vi "SLL DE AO LV2 Global.vi"(6 "AO value Array":dbl[](array[numeric]), 7 "AO Option":T2, 8 "error in (no error)":errorcluster, 9 "AO value":dbl, 10 "AO Channel Name Array":T1[](array[typedef]), 11 "AO Channel Name":T1) -> (0 "error out":errorcluster, 2 "Analog Output Array Value":dbl[](array[numeric]), 3 "Analog Output Line Value":dbl, 4 "Element Wrote":string)   [LabVIEW 2013]
uses:
  Controls/SLL DE AO Global Options.ctl
  Controls/SLL DE List of Analog Outputs.ctl
  Controls/SLL DE AO Command LV2Global Options.ctl
  Controls/SLL DE AO Min Max Range Checking Options.ctl
panel:
  out "Data Changed?":bool
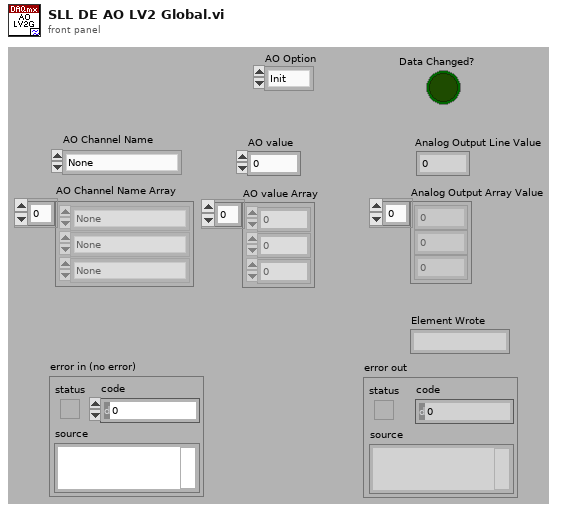
[diagram p1: front panel]
types:
  T1 = typedef "SLL DE List of Analog Outputs.ctl" = enum16{"None"}
  T2 = typedef "SLL DE AO Global Options.ctl" = enum16{"Init", "Write Line", "Write Array", "Read Line", "Read Array", "Read Full Status", "Restart AO", "Send to Safe Mode", "Stop AO"}
  T3 = typedef "SLL DE AO Command LV2Global Options.ctl" = enum16{"Init/Register Events", "Get Event Refnum", "Fire Event", "Distroy Event"}
  T4 = typedef "SLL DE AO Min Max Range Checking Options.ctl" = enum16{"Initalize Channel Range", "Check Single AO Channel", "Check Multiple AO Channels"}
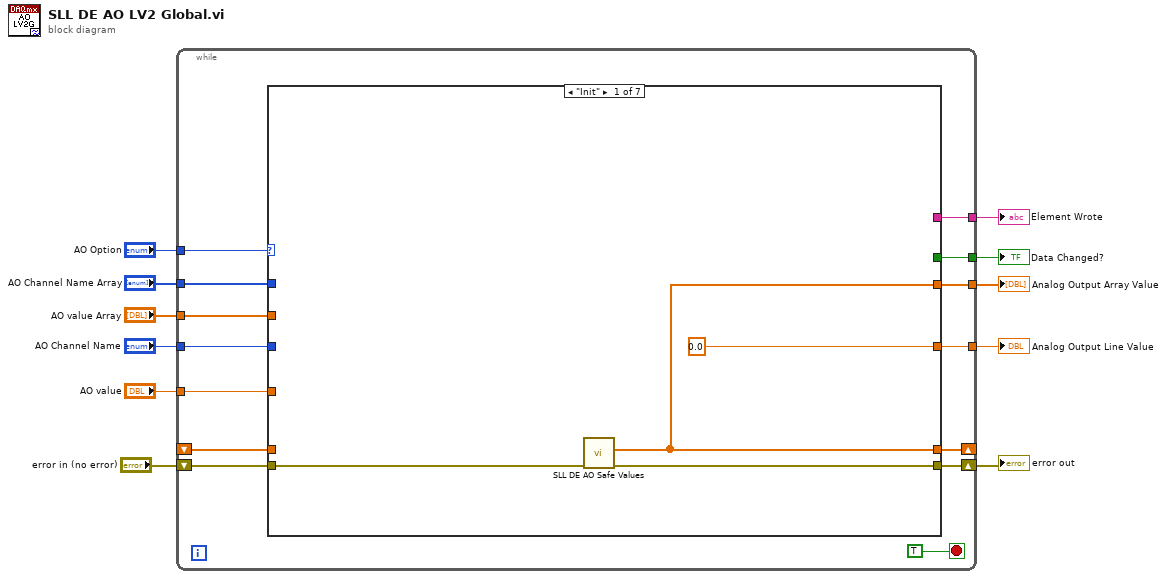
[diagram p0: block diagram]
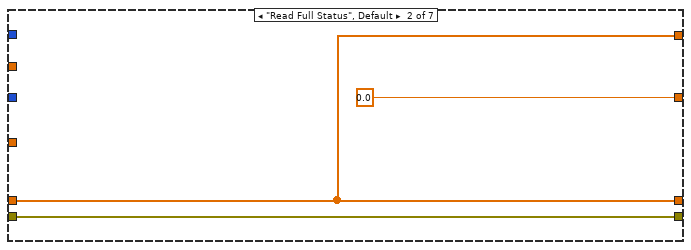
[diagram p2: hidden frame]
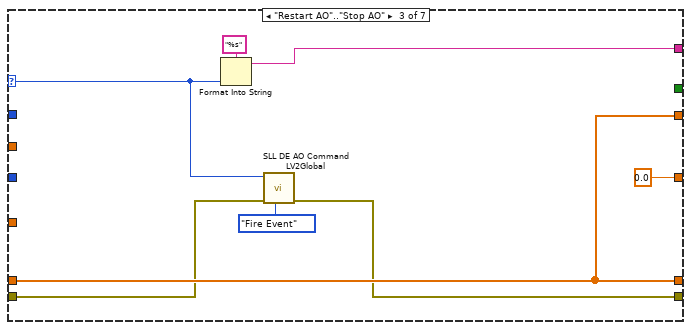
[diagram p3: hidden frame]
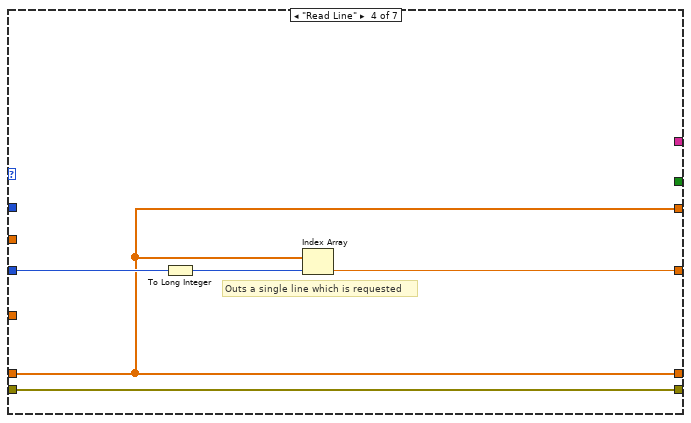
[diagram p4: hidden frame]
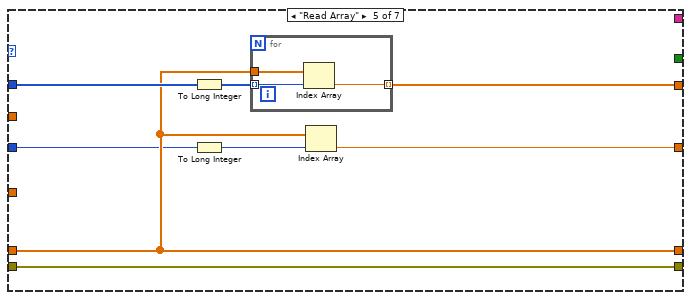
[diagram p5: hidden frame]
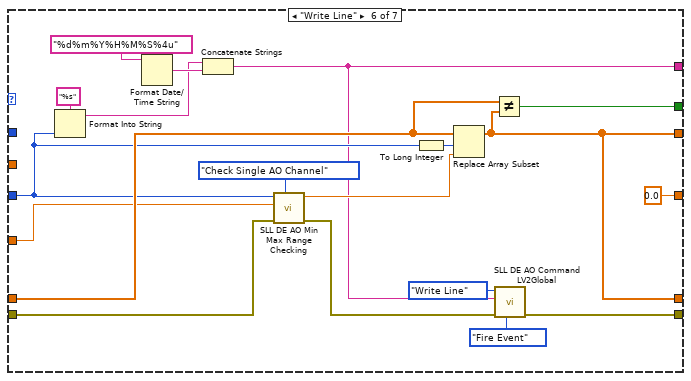
[diagram p6: hidden frame]
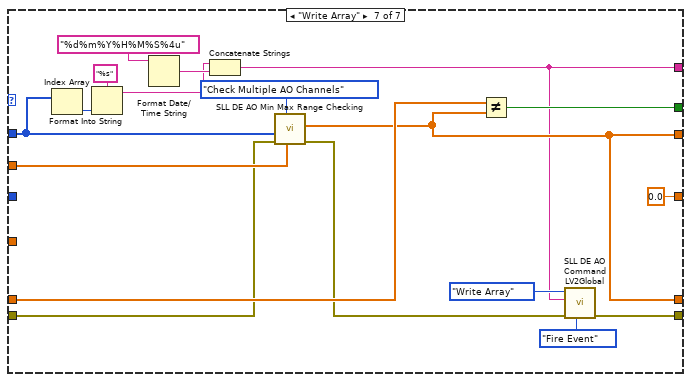
[diagram p7: hidden frame]
diagram:
  n1 = while {
    shift-right: [w24] -> _
    shift-left: _ -> [w23]
    tunnel: "AO Channel Name Array" -> [w22]
    tunnel: "AO Channel Name" -> [w21]
    tunnel: [w20] -> w9
    tunnel: [w19] -> w8
    shift-right: [w17] -> w6
    shift-left: "error in (no error)" -> [w18]
    tunnel: "AO value Array" -> [w16]
    tunnel: "AO value" -> [w15]
    tunnel: "AO Option" -> [w14]
    tunnel: [w13] -> w2
    tunnel: [w12] -> w1
    stop <- TRUE stop-if-true
    n2 = case shown="\"Init\"" w14 {
      selector: w14 -> [_ _ w35 _ _ _ _]
      tunnel: [w26 w32 w40 w43 w50 w68 w81] -> w24
      tunnel: w23 -> [_ w32 w40 w43 w50 w69 w87]
      tunnel: w22 -> [_ _ _ _ w53 _ w85]
      tunnel: w21 -> [_ _ _ w45 w49 w66 _]
      tunnel: [0.0 ("Digital Input") 0.0 ("Digital Input") 0.0 ("Digital Input") w44 w48 0.0 ("Digital Input") 0.0 ("Digital Input")] -> w20
      tunnel: [w26 w32 w40 w43 w52 w68 w81] -> w19
      tunnel: w18 -> [w28 w31 w34 w42 w51 w62 w82]
      tunnel: [w27 w31 w33 w42 w51 w60 w77] -> w17
      tunnel: w16 -> [_ _ _ _ _ _ w83]
      tunnel: w15 -> [_ _ _ _ _ w65 _]
      tunnel: [_ _ w37 _ _ w57 w76] -> w13
      tunnel: [_ _ _ _ _ w67 w86] -> w12
      frame "Init" {
        n3 = call "SLL DE AO Safe Values.vi"("error in (no error)"=w28) -> ("error out"=w27:errorcluster, "AO Safe Values"=w26:dbl[])  [unwired: 8 in, 1 out]
      }
      frame "Read Full Status", Default {
      }
      frame "Restart AO".."Stop AO" {
        n4 = Format Into String(format string="%s", w35) -> (resulting string=w37:string)  [unwired: 2 in, 1 out]
        n5 = call "SLL DE AO Command LV2Global.vi"("Option"=SLL_DE_AO_Command_LV2Global_Options."Fire Event", "Error in (no error)"=w34, "AO Option"=w35) -> ("Error out"=w33:errorcluster)  [unwired: 7 in, 1 out]
      }
      frame "Read Line" {
        # "Outs a single line which is requested"
        n6 = To Long Integer(number=w45) -> (32bit integer=w41:i32)
        n7 = Index Array(array=w43, index=w41) -> (element=w44:dbl)
      }
      frame "Read Array" {
        n8 = To Long Integer(number=w53) -> (32bit integer=w46:i32[])
        n9 = To Long Integer(number=w49) -> (32bit integer=w47:i32)
        n10 = for {
          tunnel: w50 -> [w56]
          tunnel: w46 -> [w54] mode=indexing
          tunnel: [w55] -> w52 mode=indexing
          n11 = Index Array(array=w56, index=w54) -> (element=w55:dbl)
        }
        n12 = Index Array(array=w50, index=w47) -> (element=w48:dbl)
      }
      frame "Write Line" {
        n13 = Format Into String(format string="%s", w66) -> (resulting string=w71:string)  [unwired: 2 in, 1 out]
        n14 = Format Date/Time String(time format string (%c)="%d%m%Y%H%M%S%4u") -> (date/time string=w72:string)  [unwired: 2 in]
        n15 = Concatenate Strings(w71, w72) -> (w57:string)
        n16 = call "SLL DE AO Min Max Range Checking.vi"("Option"=SLL_DE_AO_Min_Max_Range_Checking_Options."Check Single AO Channel", "error in (no error)"=w62, "AO Value"=w65, "AO Channel Name"=w66) -> ("error out"=w58:errorcluster, "AO Value Out"=w64:dbl)  [unwired: 5 in, 1 out]
        n17 = To Long Integer(number=w66) -> (32bit integer=w73:i32)
        n18 = Replace Array Subset(array=w69, new element=w64, index=w73) -> (w68:dbl[])
        n19 = Not Equal?(x=w69, y=w68) -> (x != y?=w67:bool)
        n20 = call "SLL DE AO Command LV2Global.vi"("Option"=SLL_DE_AO_Command_LV2Global_Options."Fire Event", "Error in (no error)"=w58, "Execute For"=w57, "AO Option"=SLL_DE_AO_Global_Options."Write Line") -> ("Error out"=w60:errorcluster)  [unwired: 6 in, 1 out]
      }
      frame "Write Array" {
        n21 = Index Array(array=w85) -> (element=w91:T1)  [unwired: 1 in]
        n22 = Format Into String(format string="%s", w91) -> (resulting string=w89:string)  [unwired: 2 in, 1 out]
        n23 = Format Date/Time String(time format string (%c)="%d%m%Y%H%M%S%4u") -> (date/time string=w90:string)  [unwired: 2 in]
        n24 = Concatenate Strings(w89, w90) -> (w76:string)
        n25 = call "SLL DE AO Min Max Range Checking.vi"("AO Values In"=w83, "Option"=SLL_DE_AO_Min_Max_Range_Checking_Options."Check Multiple AO Channels", "error in (no error)"=w82, "AO Channels Name"=w85) -> ("error out"=w78:errorcluster, "AO Values Out"=w81:dbl[])  [unwired: 5 in, 1 out]
        n26 = Not Equal?(x=w87, y=w81) -> (x != y?=w86:bool)
        n27 = call "SLL DE AO Command LV2Global.vi"("Option"=SLL_DE_AO_Command_LV2Global_Options."Fire Event", "Error in (no error)"=w78, "Execute For"=w76, "AO Option"=SLL_DE_AO_Global_Options."Write Array") -> ("Error out"=w77:errorcluster)  [unwired: 6 in, 1 out]
      }
    }
  }
  "error out" <- w6
  "Analog Output Line Value" <- w9
  "Analog Output Array Value" <- w8
  "Element Wrote" <- w2
  "Data Changed?" <- w1
